vi "VI Tree.vi"   [LabVIEW 2015, in "Ohaus AV Series.lvlib"]
doc: "This is the instrument driver for the Ohaus Adventurer Pro balance.\n\nThe VI Tree displays all the user-callable VIs of the instrument driver in an organized table."
uses:
  <instrlib>/Ohaus AV Series/Ohaus AV Series.lvlib
panel:
  # "(c) 2004-2009 National Instruments.  All Rights Reserved."
  # "SEE DIAGRAM\nFOR VI TREE."
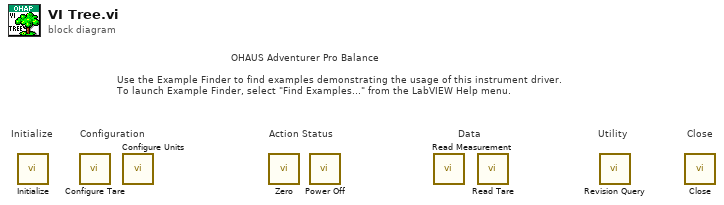
[diagram p0: block diagram]
diagram:
  # "Use the Example Finder to find examples demonstrating the usage of this instrument driver.\nTo launch Example Finder, select \"Find Examples...\" from the LabVIEW Help menu."
  # "Action Status"
  # "Data"
  # "Configuration"
  # "Utility"
  # "Close"
  # "Initialize"
  # "OHAUS Adventurer Pro Balance"
  n1 = call <instrlib>:"Initialize.vi"() -> ()  [unwired: 14 in, 2 out]
  n2 = call <instrlib>:"Configure Tare.vi"() -> ()  [unwired: 10 in, 2 out]
  n3 = call <instrlib>:"Configure Units.vi"() -> ()  [unwired: 10 in, 2 out]
  n4 = call <instrlib>:"Zero.vi"() -> ()  [unwired: 10 in, 2 out]
  n5 = call <instrlib>:"Power Off.vi"() -> ()  [unwired: 10 in, 2 out]
  n6 = call <instrlib>:"Read Measurement.vi"() -> ()  [unwired: 6 in, 6 out]
  n7 = call <instrlib>:"Read Tare.vi"() -> ()  [unwired: 8 in, 4 out]
  n8 = call <instrlib>:"Revision Query.vi"() -> ()  [unwired: 8 in, 4 out]
  n9 = call <instrlib>:"Close.vi"() -> ()  [unwired: 11 in, 1 out]
